vi "wmf_open_camera.vi"(8 "error in (no error)":errorcluster, 10 "Config path":path, 11 "camera_name":string) -> (0 "error out":errorcluster, 2 "height":i32, 3 "width":i32)   [LabVIEW 2022 SP3, in "Vision.lvlib"]
uses:
  Vision.lvlib
  <vilib>/Utility/config.llb/Read Key (I32).vi
  <vilib>/Utility/config.llb/Read Key (String).vi
  <vilib>/Utility/config.llb/NI_LVConfig.lvlib
  bin/Camera.dll
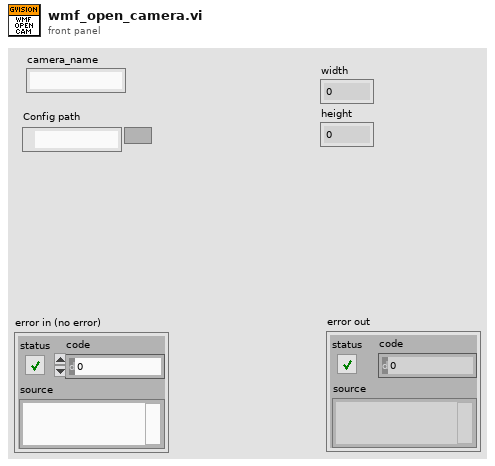
[diagram p1: front panel]
types:
  T1 = typedef "NI_LVConfig.lvlib/Config Data RefNum.ctl" = refnum<k1>
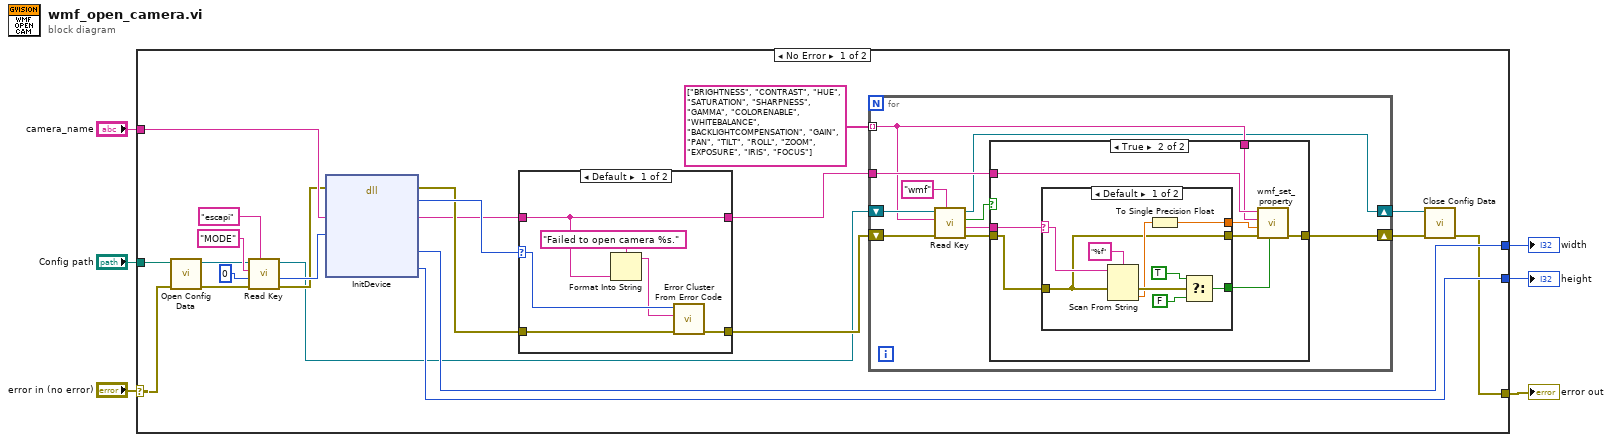
[diagram p0: block diagram]
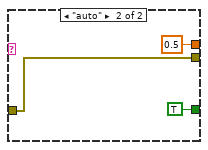
[diagram p3: hidden frame]
diagram:
  n1 = case shown="No Error" "error in (no error)" {
    selector: "error in (no error)" -> [w25 w68]
    tunnel: [w7 w68] -> w4
    tunnel: "camera_name" -> [w24 _]
    tunnel: "Config path" -> [w26 _]
    tunnel: [w23 _] -> w2
    tunnel: [w22 _] -> w1
    frame No Error {
      n2 = call <vilib>:"Open Config Data.vi"("error in (no error)"=w25, "configuration file path"=w26) -> ("error out"=w15:errorcluster, "refnum"=w18:T1)  [unwired: 7 in, 1 out]
      n3 = call-poly <vilib>:"Read Key.vi"("section"="escapi", "error in (no error)"=w15, "default value"=0, "key"="MODE", "refnum"=w18) -> ("error out"=w16:errorcluster, "value"=w17:i32, "refnum out"=w10:T1)  [unwired: 3 in, 1 out]
      n4 = dll-call lib="C:/Users/Caleb/Desktop/nebraska-silicon-lab/pixel-gantry-extra/LV/bin/Camera.dll" fn="InitDevice"(error in=w16, "camera_name"=w24, "mode_id"=w17) -> (error out=w27:errorcluster, "return type"=w28:i32, "camera_name"=w14:string, "width"=w23:i32, "height"=w22:i32)  [unwired: 5 in, 1 out]
      n5 = case shown="Default" w28 {
        selector: w28 -> [w63 _]
        tunnel: w27 -> [w65 w67]
        tunnel: [w64 w67] -> w12
        tunnel: w14 -> [w60 w66]
        tunnel: [w60 w66] -> w11
        frame Default {
          n6 = Format Into String(format string="Failed to open camera %s." ("error message (\"\")"), w60) -> (resulting string=w61:string)  [unwired: 2 in, 1 out]
          n7 = call <vilib>:"Error Cluster From Error Code.vi"("error in (no error)"=w65, "error message (\"\")"=w61, "error code (0)"=w63) -> ("error out"=w64:errorcluster)  [unwired: 6 in]
        }
        frame 0 {
        }
      }
      n8 = for {
        tunnel: string[] ["BRIGHTNESS", "CONTRAST", "HUE", "SATURATION", "SHARPNESS", "GAMMA", "COLORENABLE", "WHITEBALANCE", "BACKLIGHTCOMPENSATION", "GAIN", "PAN", "TILT", "ROLL", "ZOOM", "EXPOSURE", "IRIS", "FOCUS"] -> [w31] mode=indexing
        shift-right: [w30] -> w9
        shift-left: w10 -> [w38]
        shift-right: [w33] -> w8
        shift-left: w12 -> [w36]
        tunnel: w11 -> [w32]
        n9 = call-poly <vilib>:"Read Key.vi"("section"="wmf", "error in (no error)"=w36, "key"=w31, "refnum"=w38) -> ("error out"=w34:errorcluster, "value"=w35:string, "found?"=w29:bool, "refnum out"=w30:T1)  [unwired: 4 in]
        n10 = case shown="True" w29 {
          tunnel: w35 -> [_ w47]
          tunnel: w34 -> [w39 w46]
          tunnel: [w39 w44] -> w33
          tunnel: w32 -> [_ w43]
          tunnel: w31 -> [_ w42]
          frame False {
          }
          frame True {
            n11 = case shown="Default" w47 {
              selector: w47 -> [w56 _]
              tunnel: [w51 TRUE] -> w40
              tunnel: [w54 sgl 0.5] -> w41
              tunnel: w46 -> [w50 w59]
              tunnel: [w50 w59] -> w45
              frame Default {
                n12 = Scan From String(format string="%f", input string=w56, error in=w50) -> (error out=w53:errorcluster, output 1=w52:dbl)  [unwired: 2 in, 2 out]
                n13 = To Single Precision Float(number=w52) -> (single precision float=w54:sgl)
                n14 = Select(t=TRUE, s=w53, f=FALSE) -> (s? t:f=w51:bool)
              }
              frame "auto" {
              }
            }
            n15 = call "wmf_set_property.vi"("Auto"=w40, "error in (no error)"=w45, "Value"=w41, "property name"=w42, "camera_name"=w43) -> ("error out"=w44:errorcluster)  [unwired: 6 in]
          }
        }
      }
      n16 = call <vilib>:"Close Config Data.vi"("error in (no error)"=w8, "refnum"=w9) -> ("error out"=w7:errorcluster)  [unwired: 8 in, 1 out]
    }
    frame Error {
    }
  }
  "error out" <- w4
  "width" <- w2
  "height" <- w1
